vi "Mul 12 (Async).vi"() -> (0 "error out":errorcluster, 2 "Mul 12 Promise":refnum<class "Promise.lvclass">)   [LabVIEW 2020, in "Futures-Examples.lvlib"]
uses:
  Futures-Examples.lvlib
  Promises/Promise/Promise.lvclass
  DoubleValue/DoubleValue.lvclass
  C:/dev/lv/2020/lv-promises/Promises/Value/Value.lvclass
  Mul 12 Task.vi
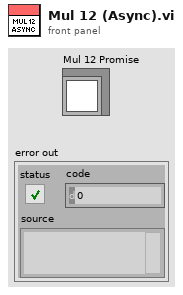
[diagram p1: front panel]
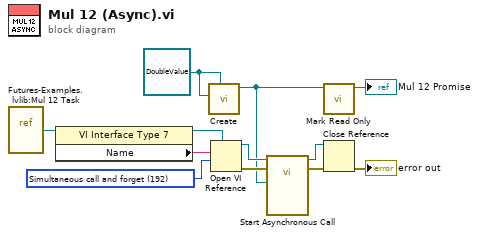
[diagram p0: block diagram]
diagram:
  w6 = 192 items=["Record modifications"=1, "Open templates for editing"=2, "Prompt user to save"=4, "Prepare for reentrant run"=8, "Prompt to find missing subVIs"=16, "Hide loading dialog box"=32, "Enable simultaneous calls"=64, "Prepare to call and forget"=128, "Simultaneous call and forget"=192, "Prepare to call and collect"=256, "Simultaneous call and collect"=320]
  w12 = refnum<class "DoubleValue.lvclass"> refnum ("Futures-Examples.lvlib:DoubleValue.lvclass")
  n1 = vi-ref "Futures-Examples.lvlib:Mul 12 Task.vi"() -> (w4:refnum<vi>)
  n2 = property class="VI Interface Type 7"(reference=w4) -> (reference out=w7:refnum<vi>, "Name"=w5:string)  [unwired: 1 in, 1 out]
  n3 = call "Create.vi"("Param Type (None)"=w12, "Result Type"=w12) -> ("Promise"=w3:refnum<class "Promise.lvclass">)  [unwired: 8 in, 1 out]
  n4 = Open VI Reference(type specifier VI Refnum (for type only)=w7, vi path=w5, options=w6) -> (vi reference=w9:refnum<vi>, error out=w8:errorcluster)  [unwired: 3 in]
  n5 = call-by-ref "Start Asynchronous Call"(reference=w9, error in=w8, "Promise"=w3) -> (reference out=w11:refnum<vi>, error out=w10:errorcluster)  [unwired: 11 in]
  n6 = call "Mark Read Only.vi"("Promise in"=w3) -> ("Promise out"=→"Mul 12 Promise":refnum<class "Promise.lvclass">)  [unwired: 9 in, 1 out]
  n7 = Close Reference(reference=w11, error in (no error)=w10) -> (error out=→"error out":errorcluster)
